vi "Config.vi"(7 "LabVIEW Web Service Request":refnum<class "Web Request.lvclass">) -> ()   [LabVIEW 2021]
uses:
  <vilib>/wsapi/Web Request.lvclass
panel:
  out "postdata":string
  out "UploadedFilesList":T1(array[cluster])
  # "Use the Web Service Request input terminal to call the VIs on the Web Services palette. Do not remove it from the connector pane unless you don't need access to the palette."
  # "Each additional control wired to the connector pane will be available as an input in the URL. To include an indicator in terminal-mode output (the default setting), it must also be wired to the connector pane."
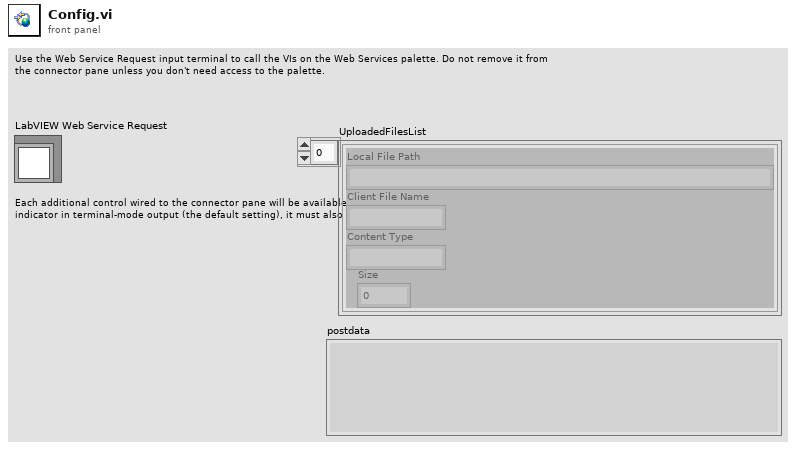
[diagram p1: front panel]
types:
  T1 = cluster{"Local File Path":string, "Client File Name":string, "Content Type":string, "Size":u32}[]
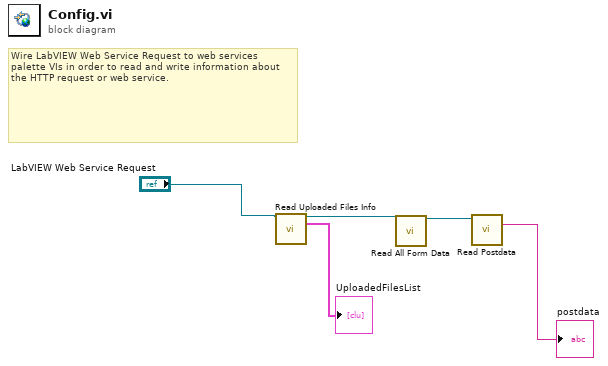
[diagram p0: block diagram]
diagram:
  # "Wire LabVIEW Web Service Request to web services palette VIs in order to read and write information about the HTTP request or web service."
  n1 = call <vilib>:"Read Uploaded Files Info.vi"("LabVIEW Web Service Request"="LabVIEW Web Service Request") -> ("LabVIEW Web Service Request out"=w3:refnum<class "Web Request.lvclass">, "UploadedFilesList"=→"UploadedFilesList":T1)  [unwired: 12 in, 1 out]
  n2 = call <vilib>:"Read All Form Data.vi"("LabVIEW Web Service Request"=w3) -> ("LabVIEW Web Service Request out"=w2:refnum<class "Web Request.lvclass">)  [unwired: 10 in, 4 out]
  n3 = call <vilib>:"Read Postdata.vi"("LabVIEW Web Service Request"=w2) -> ("postdata"=→"postdata":string)  [unwired: 12 in, 2 out]
